vi "Unibot - Nonlinear Model 2.vi"() -> (0 "xPos1":dbl=-0.3578561321200968, 1 "alpha1":dbl=0.11676928692181643, 3 "states":dbl[](array[numeric])=[0.11676928692181643, -0.3578561321200968, -0.19175807659191071, 0.3912657493379608])   [LabVIEW 2012]
uses:
  <vilib>/Simulation/Implementation/Shared/SIMSCR Execution Mode.ctl
  <vilib>/Simulation/Scripting/Companion Diagram/SimConfigNode/SimParams.ctl
  <vilib>/Simulation/Scripting/Companion Diagram/SimConfigNode/_simSolvers.ctl
  <vilib>/Simulation/Param Hierarchy/Typedefs/SIMPH Param Control Actions.ctl
  <vilib>/Simulation/Implementation/Shared/SIM limit type.ctl
  <vilib>/Simulation/Implementation/Shared/NILVSim_ParamChanged.vi
  <vilib>/Simulation/ContinuousLinear/Implementation/NILVSim Integrator new.llb/SIM Integrator distributor (scalar).vi
  <vilib>/Simulation/ContinuousLinear/Implementation/NILVSim Integrator new.llb/SIM Integrator collector (scalar).vi
  <vilib>/Simulation/Implementation/Shared/NILVSim_Manager.vi
  <vilib>/Simulation/Implementation/Shared/NILVSim_FinalizeModel.vi
  <vilib>/Simulation/Implementation/Shared/SIM Unbundle Sim Info.vi
  <vilib>/Utility/error.llb/Clear Errors.vi
  <vilib>/Simulation/Implementation/Shared/NILVSim_GetModelError.vi
  <vilib>/Simulation/Implementation/Shared/SIM SimErrorHandler.vi
  <vilib>/Simulation/Implementation/Shared/SIM Bundle Sim Info.vi
  <vilib>/Simulation/Implementation/Shared/SIMSH Read Queue.vi
  <vilib>/Simulation/Implementation/Shared/NILVSim_Initialize.vi
  <vilib>/Simulation/Utility/Implementation/NILVSim Get Time and IsAcceptedStep.vi
  <vilib>/Simulation/Scripting/Companion Diagram/SimConfigNode/SimDog.xnode
  <vilib>/Simulation/Implementation/XNodeFramework/SimXNode/SimX.xnode
  <vilib>/Simulation/ContinuousLinear/Implementation/NILVSim Integrator new.llb/SIM Integrator (scalar).vi
  <vilib>/ptbypt/NI_PtbyPt.lvlib
  <vilib>/Simulation/Implementation/Shared/NI_SIM_Implementation.lvlib
panel:
  in  "initial x position":dbl
  in  "initial x velocity":dbl
  in  "initial velocity alpha":dbl
  in  "Moment of Inetia of the frame wrt to center of mass (Ifg)":dbl=20.0
  in  "Distance from center of wheel to center of mass (Rf)":dbl=0.463
  in  "Mass of Frame (mf)":dbl=25.0
  in  "Amplifier Gain":dbl(slide)=1.0 scale=0.0..0.1
  in  "initial alpha":dbl=3.14159
  in  "Torque (Tau)":dbl=1.0
  # "Legend: \nC.G.  - Center of Gravity\nl       - Length (m)\nJ      - Moment of Inertia (kg(m^2)\nM     - Mass (kg)"
  # "Derived Parameters"
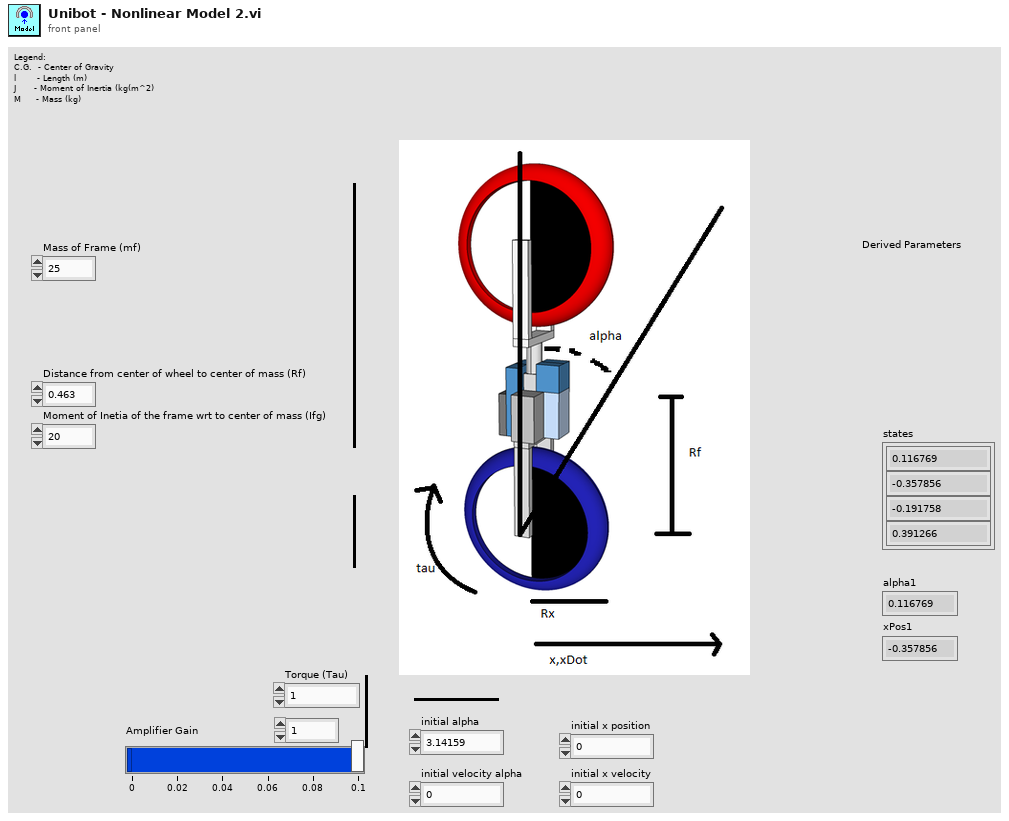
[diagram p1: front panel]
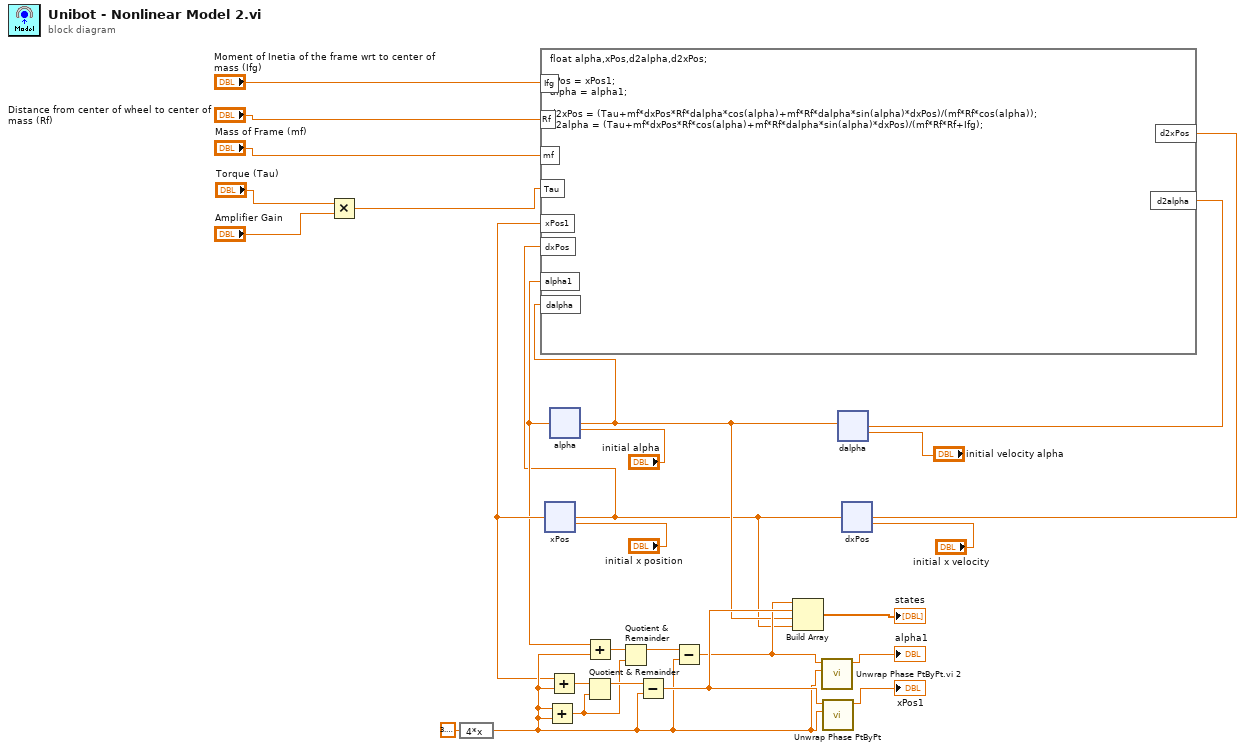
[diagram p0: block diagram]
diagram:
  n1 = Multiply ("Multiply 8")(x="Torque (Tau)", y="Amplifier Gain") -> (x*y=w23:dbl)
  n2 = expression code="4*x"(3.141592653589793 ("Constant")) -> (w10:dbl)
  n3 = Add ("Add 6")(x=w10, y=w10) -> (x+y=w14:dbl)
  n4 = formula code="float alpha,xPos,d2alpha,d2xPos;\n\nxPos = xPos1;\nalpha = alpha1;\n\nd2xPos = (Tau+mf*dxPos*Rf*dalpha*cos(alpha)+mf*Rf*dalpha*sin(alpha)*dxPos)/(mf*Rf*cos(alpha));\nd2alpha = (Tau+mf*dxPos*Rf*cos(alpha)+mf*Rf*dalpha*sin(alpha)*dxPos)/(mf*Rf*Rf+Ifg);" ("Formula Node 2")("Ifg"="Moment of Inetia of the frame wrt to center of mass (Ifg)", "Rf"="Distance from center of wheel to center of mass (Rf)", "mf"="Mass of Frame (mf)", "Tau"=w23, "alpha1"=w2, "dalpha"=w7, "dxPos"=w1, "xPos1"=w3) -> ("d2alpha"=w22:dbl, "d2xPos"=w6:dbl)
  n5 = xnode "dalpha"("input"=w22, "initial condition"="initial velocity alpha") -> ("output"=w7:dbl)  [unwired: 8 in, 2 out]
  n6 = xnode "alpha"("input"=w7, "initial condition"="initial alpha") -> ("output"=w2:dbl)  [unwired: 8 in, 2 out]
  n7 = Add ("Add 5")(x=w2, y=w10) -> (x+y=w16:dbl)
  n8 = Quotient & Remainder ("Quotient & Remainder 2")(x=w16, y=w14) -> (x-y*floor(x/y)=w17:dbl)  [unwired: 1 out]
  n9 = Subtract ("Subtract 2")(x=w17, y=w10) -> (x-y=w8:dbl)
  n10 = call "Unwrap Phase PtByPt.vi 2"("wrap base"=w10, "phase"=w8) -> ("unwrapped phase"=→"alpha1":dbl)  [unwired: 9 in]
  n11 = xnode "dxPos"("input"=w6, "initial condition"="initial x velocity") -> ("output"=w1:dbl)  [unwired: 8 in, 2 out]
  n12 = xnode "xPos"("input"=w1, "initial condition"="initial x position") -> ("output"=w3:dbl)  [unwired: 8 in, 2 out]
  n13 = Add ("Add 4")(x=w3, y=w10) -> (x+y=w19:dbl)
  n14 = Quotient & Remainder(x=w19, y=w14) -> (x-y*floor(x/y)=w18:dbl)  [unwired: 1 out]
  n15 = Subtract(x=w18, y=w10) -> (x-y=w13:dbl)
  n16 = Build Array(w8, w13, w7, w1) -> (→"states":dbl[])
  n17 = call <vilib>:"Unwrap Phase PtByPt.vi"("wrap base"=w10, "phase"=w13) -> ("unwrapped phase"=→"xPos1":dbl)  [unwired: 9 in]
